vi "ziExample-UHFLI-ConnectDevice.vi"() -> ()   [LabVIEW 2009]
doc: "Control a Zurich instrument device via the LabOne Labview API. \nRequirements: Zurich Instruments UHFLI \nThis example VI connects and disconnects UHF instruments to a data server using different interfaces.\n\n© Zurich Instruments AG, www.zhinst.com"
uses:
  <vilib>/Utility/error.llb/DialogType.ctl
  <instrlib>/Zurich Instruments LabOne/Zurich Instruments LabOne.lvlib
panel:
  in  "Address":string="localhost:8004"
  in  "Selected Device":i32(listbox)
  in  "Device Interface":string(combo)
  in  "Interface Params (\"\")":string
  in  "DisConnectDevice":bool
  in  "ConnectDevice":bool
  in  "Available Devices":i32(listbox)
  in  "Update":bool
  in  "Stop":bool
  out "Error Out":errorcluster
  # "Tested Instruments:\n- UHFLI"
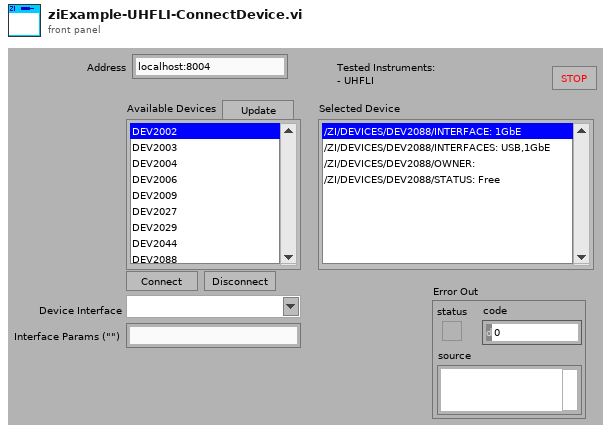
[diagram p1: front panel]
types:
  T1 = typedef "Zurich Instruments LabOne.lvlib/ziTypeHandle.ctl" = cluster{"handleValid":bool, "Conn":u64, "Path Prefix":string, "Handle":u64, "Connected":bool, "Clockbase(s)":dbl}
  T2 = typedef "DialogType.ctl" = u16
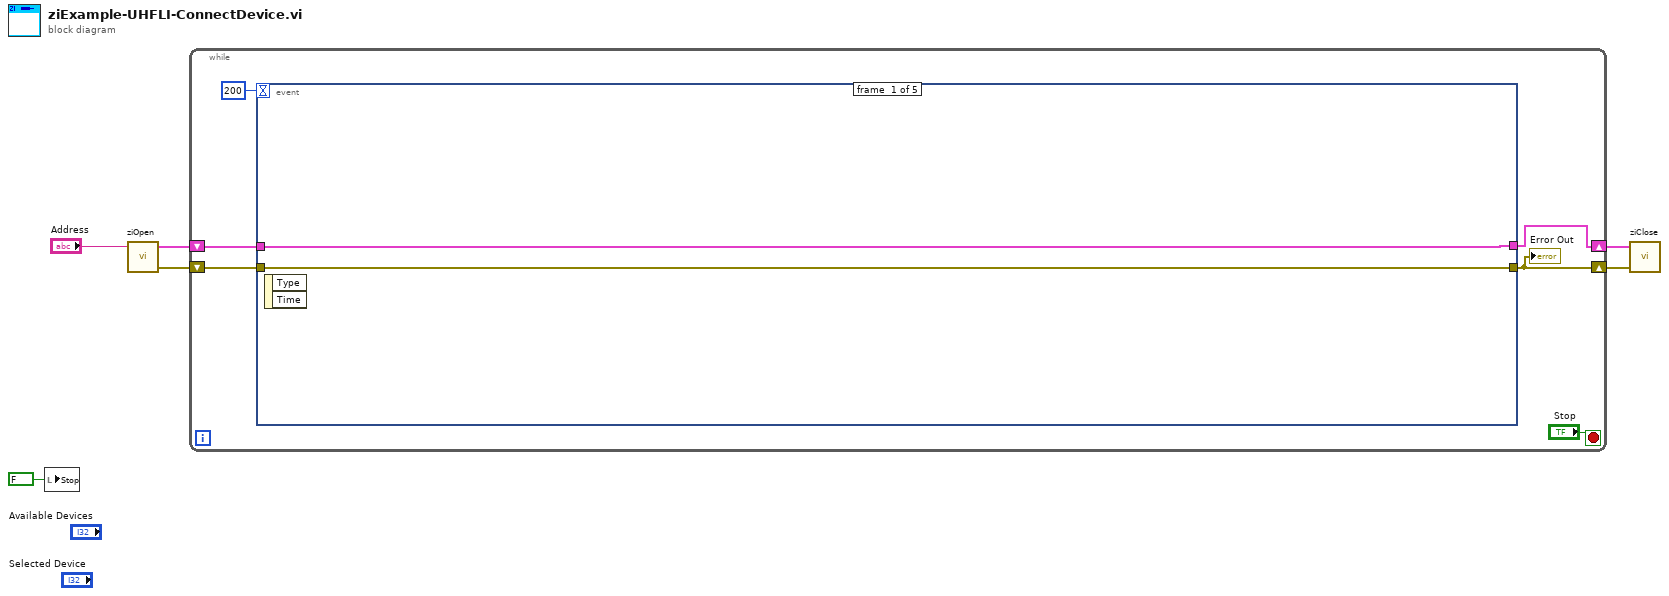
[diagram p0: block diagram]
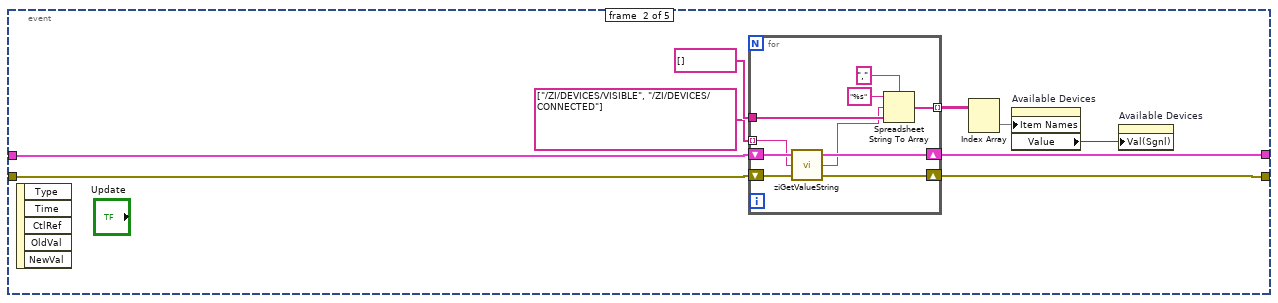
[diagram p2: hidden frame]
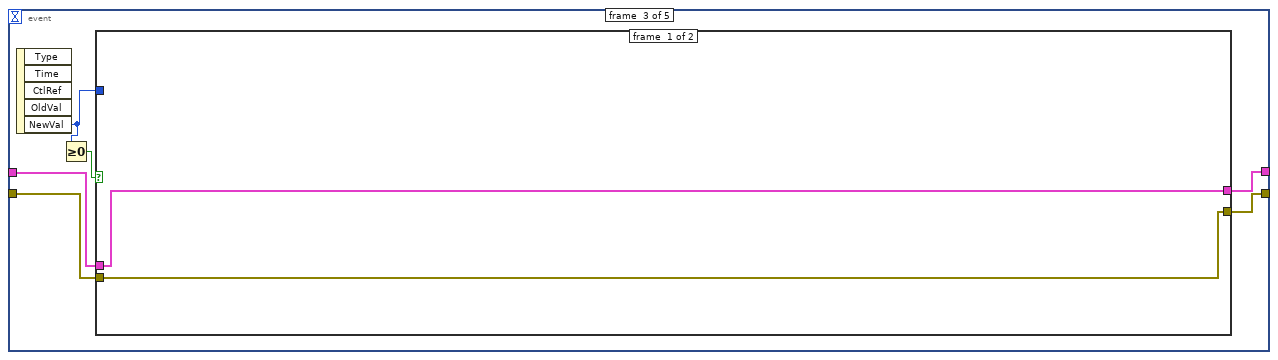
[diagram p3: hidden frame]
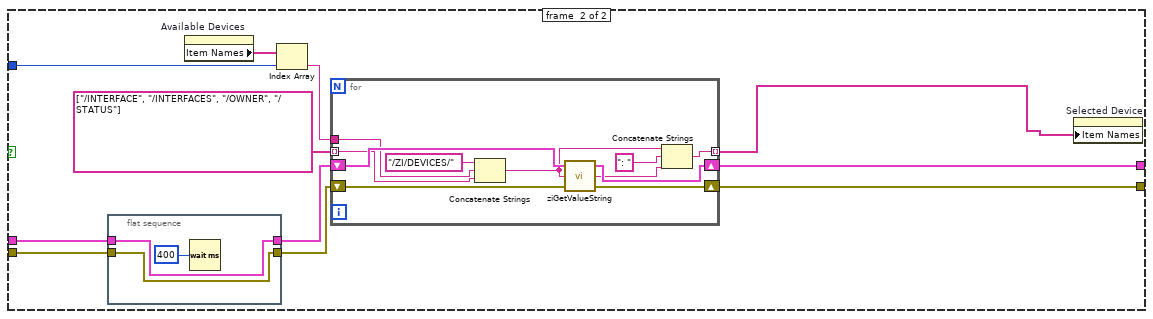
[diagram p4: hidden frame]
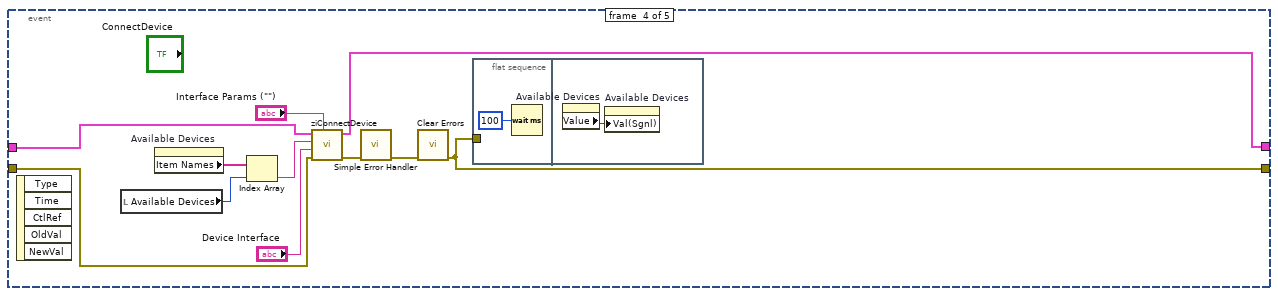
[diagram p5: hidden frame]
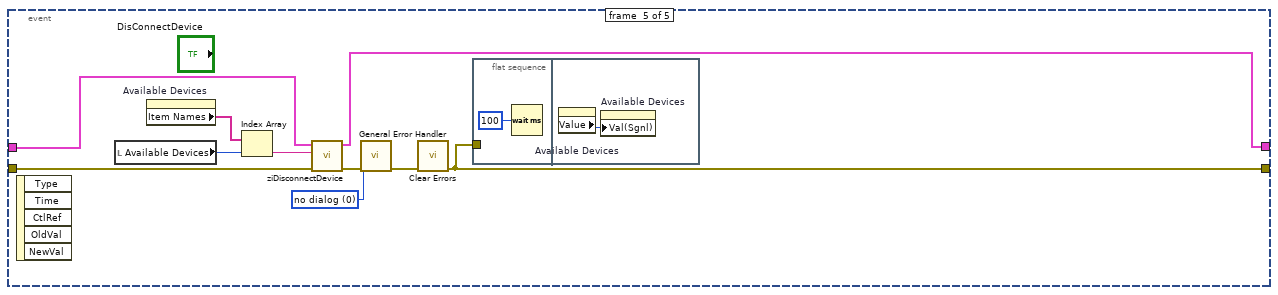
[diagram p6: hidden frame]
diagram:
  n1 = local write "Stop"(FALSE ("Stop")) -> ()
  n2 = call <instrlib>:"ziOpen.vi"("Address"="Address") -> ("Error Out"=w2:errorcluster, "HandleOut"=w3:T1)  [unwired: 1 in, 3 out]
  n3 = while {
    shift-right: [w9] -> w6
    shift-left: w3 -> [w11]
    shift-right: [w8] -> w5
    shift-left: w2 -> [w10]
    stop <- "Stop" stop-if-true
    n4 = event shown="[1] \"Update\": Value Change" {
      selector: _ -> [_ _ _ _ _]
      dyn-events: _ -> [_ _ _ _ _]
      timeout: 200 -> [_ _ _ _ _]
      tunnel: w11 -> [w14 w16 w38 w76 w88]
      tunnel: w10 -> [w13 w15 w39 w75 w87]
      tunnel: [w14 w21 w37 w77 w89] -> w9
      tunnel: [w13 w23 w36 w67 w81] -> w8
      event #0 {
        n5 = event-data() -> ()  [unwired: 1 in, 2 out]
      }
      event #1 {
        n6 = event-data() -> ()  [unwired: 1 in, 5 out]
        n7 = for {
          shift-right: [w30] -> w21
          shift-left: w16 -> [w31]
          shift-right: [w32] -> w23
          shift-left: w15 -> [w33]
          tunnel: string[] [] ("array") -> [w27]
          tunnel: [w26] -> w18 mode=indexing
          tunnel: string[] ["/ZI/DEVICES/VISIBLE", "/ZI/DEVICES/CONNECTED"] -> [w24] mode=indexing
          n8 = call <instrlib>:"ziGetValueString.vi"("error in"=w33, "Path"=w24, "Handle In"=w31) -> ("error out"=w32:errorcluster, "Value"=w25:string, "Handle Out"=w30:T1)
          n9 = Spreadsheet String To Array(delimiter (Tab)=",", format string="%s", spreadsheet string=w25, array type (2D Dbl)=w27) -> (array=w26:string[])
        }
        n10 = Index Array(array=w18) -> (element=w19:string[])  [unwired: 2 in]
        n11 = property on="Available Devices" class="LstBox (strict)"("Item Names"=w19) -> ("Value"=w17:i32)  [unwired: 2 in, 2 out]
        n12 = property on="Available Devices" class="LstBox (strict)"("Val(Sgnl)"=w17) -> ()  [unwired: 2 in, 2 out]
      }
      event #2 {
        n13 = event-data() -> ("NewVal"=w34:i32)  [unwired: 1 in, 4 out]
        n14 = Greater Or Equal To 0?(x=w34) -> (x >= 0?=w35:bool)
        n15 = case shown="True" w35 {
          tunnel: w34 -> [_ w48]
          tunnel: w39 -> [w40 w47]
          tunnel: w38 -> [w41 w46]
          tunnel: [w41 w44] -> w37
          tunnel: [w40 w43] -> w36
          frame #0 {
          }
          frame #1 {
            n16 = flat-sequence {
              tunnel: w46 -> [w54]
              tunnel: w47 -> [w55]
              tunnel: [w55] -> w51
              tunnel: [w54] -> w50
              frame #0 {
                n17 = Wait (ms)(milliseconds to wait=u32 400) -> ()  [unwired: 1 out]
              }
            }
            n18 = property on="Available Devices" class="LstBox (strict)"() -> ("Item Names"=w49:string[])  [unwired: 2 in, 2 out]
            n19 = Index Array(array=w49, index=w48) -> (element=w45:string)
            n20 = for {
              tunnel: string[] ["/INTERFACE", "/INTERFACES", "/OWNER", "/STATUS"] -> [w59] mode=indexing
              shift-right: [w65] -> w44
              shift-left: w50 -> [w66]
              tunnel: [w64] -> w42 mode=indexing
              shift-right: [w62] -> w43
              shift-left: w51 -> [w63]
              tunnel: w45 -> [w57]
              n21 = Concatenate Strings("/ZI/DEVICES/" ("string"), w57, w59) -> (w56:string)
              n22 = call <instrlib>:"ziGetValueString.vi"("error in"=w63, "Path"=w56, "Handle In"=w66) -> ("error out"=w62:errorcluster, "Value"=w61:string, "Handle Out"=w65:T1)
              n23 = Concatenate Strings(w56, ": " ("string"), w61) -> (w64:string)
            }
            n24 = property on="Selected Device" class="LstBox (strict)"("Item Names"=w42) -> ()  [unwired: 2 in, 2 out]
          }
        }
      }
      event #3 {
        n25 = event-data() -> ()  [unwired: 1 in, 5 out]
        n26 = local read "Available Devices"() -> (w70:i32)
        n27 = property on="Available Devices" class="LstBox (strict)"() -> ("Item Names"=w72:string[])  [unwired: 2 in, 2 out]
        n28 = Index Array(array=w72, index=w70) -> (element=w71:string)
        n29 = call <instrlib>:"ziConnectDevice.vi"("Device Interface Params (\"\")"="Interface Params (\"\")", "Error In"=w75, "Device Interface"="Device Interface", "Device Serial"=w71, "Handle In"=w76) -> ("Error Out"=w74:errorcluster, "Handle Out"=w77:T1)  [unwired: 5 in]
        n30 = call <vilib>:"Simple Error Handler.vi"("error in (no error)"=w74) -> ("error out"=w68:errorcluster)  [unwired: 4 in, 4 out]
        n31 = call <vilib>:"Clear Errors.vi"("error in (no error)"=w68) -> ("error out"=w67:errorcluster)  [unwired: 6 in]
        n32 = flat-sequence {
          tunnel: w67 -> [_]
          frame #0 {
            n33 = Wait (ms)(milliseconds to wait=u32 100) -> ()  [unwired: 1 out]
          }
          frame #1 {
            n34 = property on="Available Devices" class="LstBox (strict)"() -> ("Value"=w79:i32)  [unwired: 2 in, 2 out]
            n35 = property on="Available Devices" class="LstBox (strict)"("Val(Sgnl)"=w79) -> ()  [unwired: 2 in, 2 out]
          }
        }
      }
      event #4 {
        w80 = T2 0 items=["no dialog", "OK message", "continue or stop message", "OK message + warnings", "continue/stop + warnings"] ("type of dialog (OK msg:1)")
        n36 = event-data() -> ()  [unwired: 1 in, 5 out]
        n37 = local read "Available Devices"() -> (w84:i32)
        n38 = property on="Available Devices" class="LstBox (strict)"() -> ("Item Names"=w86:string[])  [unwired: 2 in, 2 out]
        n39 = Index Array(array=w86, index=w84) -> (element=w85:string)
        n40 = call <instrlib>:"ziDisconnectDevice.vi"("Error In"=w87, "Device Serial"=w85, "Handle In"=w88) -> ("Error Out"=w82:errorcluster, "Handle Out"=w89:T1)  [unwired: 7 in]
        n41 = call <vilib>:"General Error Handler.vi"("type of dialog (OK msg:1)"=w80, "error in (no error)"=w82) -> ("error out"=w83:errorcluster)  [unwired: 9 in, 4 out]
        n42 = call <vilib>:"Clear Errors.vi"("error in (no error)"=w83) -> ("error out"=w81:errorcluster)  [unwired: 6 in]
        n43 = flat-sequence {
          tunnel: w81 -> [_]
          frame #0 {
            n44 = Wait (ms)(milliseconds to wait=u32 100) -> ()  [unwired: 1 out]
          }
          frame #1 {
            n45 = property on="Available Devices" class="LstBox (strict)"() -> ("Value"=w91:i32)  [unwired: 2 in, 2 out]
            n46 = property on="Available Devices" class="LstBox (strict)"("Val(Sgnl)"=w91) -> ()  [unwired: 2 in, 2 out]
          }
        }
      }
    }
    "Error Out" <- w8
  }
  n47 = call <instrlib>:"ziClose.vi"("Error In"=w5, "Handle In"=w6) -> ()  [unwired: 4 out]
